vi "Set COMM Address.vi"(8 "error in (no error)":errorcluster, 10 "COMM Address":string, 11 "Hardware in":refnum<class "Hardware.lvclass">) -> (0 "error out":errorcluster, 3 "Hardware out":refnum<class "Hardware.lvclass">)   [LabVIEW 2016, in "Hardware.lvlib" / "Hardware.lvclass"]
uses:
  <userlib>/Common Components/Hardware/Abstract Hardware/Hardware.lvclass
  <userlib>/Common Components/Hardware/Abstract Hardware/Hardware.lvclass/Hardware.ctl
  <userlib>/Common Components/Hardware/DevInfo/DevInfo.lvclass/DevInfo.ctl
  <userlib>/Common Components/Hardware/Abstract Hardware/Read DevInfo.vi
  <userlib>/Common Components/Hardware/DevInfo/Write COMM Address.vi
  <userlib>/Common Components/Hardware/DevInfo/DevInfo.lvclass
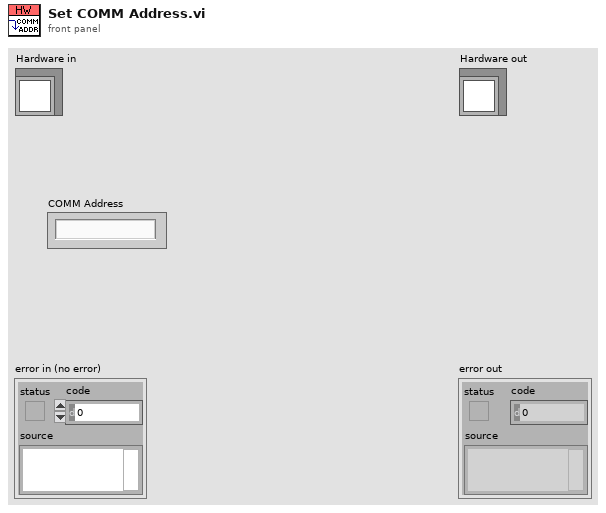
[diagram p1: front panel]
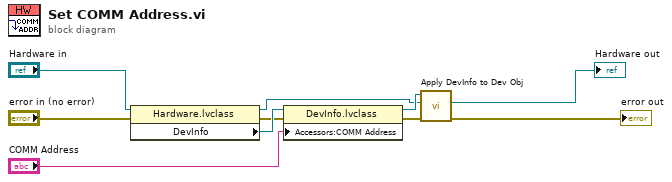
[diagram p0: block diagram]
diagram:
  n1 = property class="Hardware.lvclass"(reference="Hardware in", error in="error in (no error)") -> (reference out=w5:refnum<class "Hardware.lvclass">, error out=w2:errorcluster, "DevInfo"=w8:refnum<class "DevInfo.lvclass">)
  n2 = property class="DevInfo.lvclass"(reference=w8, error in=w2, "Accessors:COMM Address"="COMM Address") -> (reference out=w6:refnum<class "DevInfo.lvclass">, error out=w1:errorcluster)
  n3 = call <userlib>:"Apply DevInfo to Dev Obj.vi"("error in (no error)"=w1, "Dev Obj in"=w5, "DevInfo in"=w6) -> ("error out"=→"error out":errorcluster, "Dev Obj out"=→"Hardware out":refnum<class "Hardware.lvclass">)  [unwired: 6 in, 1 out]
